vi "Initialize Stimulator_v0.vi"(4 "error in (no error)":errorcluster, 6 "Initialization Parameters":T6={"Stimulator Control"={"Name"="", "Mode"=enum."SIM", "Visa Timeout"=0}, "Initialization Parameters"={"Frequency"=0.0, "N Factor"=0, "D/T Int"=0.0, "Active Channels"=[TRUE, TRUE, TRUE, TRUE, TRUE], "LF Channels"=[FALSE, FALSE, FALSE, FALSE, FALSE]}}, 7 "Stimulator":T1={"Log File In"=refnum, "Stimulator In"="", "Stimulator Mode"="", "Log Data"=FALSE, "Doublet/Triplet  Interval"=0.0, "Stim Frequency"=0.0, "N-Factor"=0, "Active Channels"=[], "Low-Frequency Channels"=[], "Stimulator State"=enum."Closed", "Mode Array"=[], "Current Array"=[], "Pulse Duration Array"=[], "VISA Timeout"=50}) -> (0 "error out":errorcluster, 1 "Write to Log":string, 2 "Response":u8, 3 "Stimulator Out":T1={"Log File In"=refnum, "Stimulator In"="", "Stimulator Mode"="", "Log Data"=FALSE, "Doublet/Triplet  Interval"=0.0, "Stim Frequency"=40.0, "N-Factor"=0, "Active Channels"=[TRUE, TRUE, TRUE, TRUE, TRUE], "Low-Frequency Channels"=[FALSE, FALSE, FALSE, FALSE, FALSE], "Stimulator State"=enum."Closed", "Mode Array"=[], "Current Array"=[], "Pulse Duration Array"=[], "VISA Timeout"=50})   [LabVIEW 2019]
doc: "Use this template to build a VI to use as a subVI."
uses:
  Controls/Stimulator Cluster.ctl
  Controls/Stimulator Mode.ctl
  Version 2/Data Type Defs/Pulse Mode (array).ctl
  Controls/Stim Current Array.ctl
  Controls/Pulse Duration Array.ctl
  Version 2/Data Type Defs/Obsolete/Stimulator Init Control_obs.ctl
  Version 2/Data Type Defs/Stim Init Data.ctl
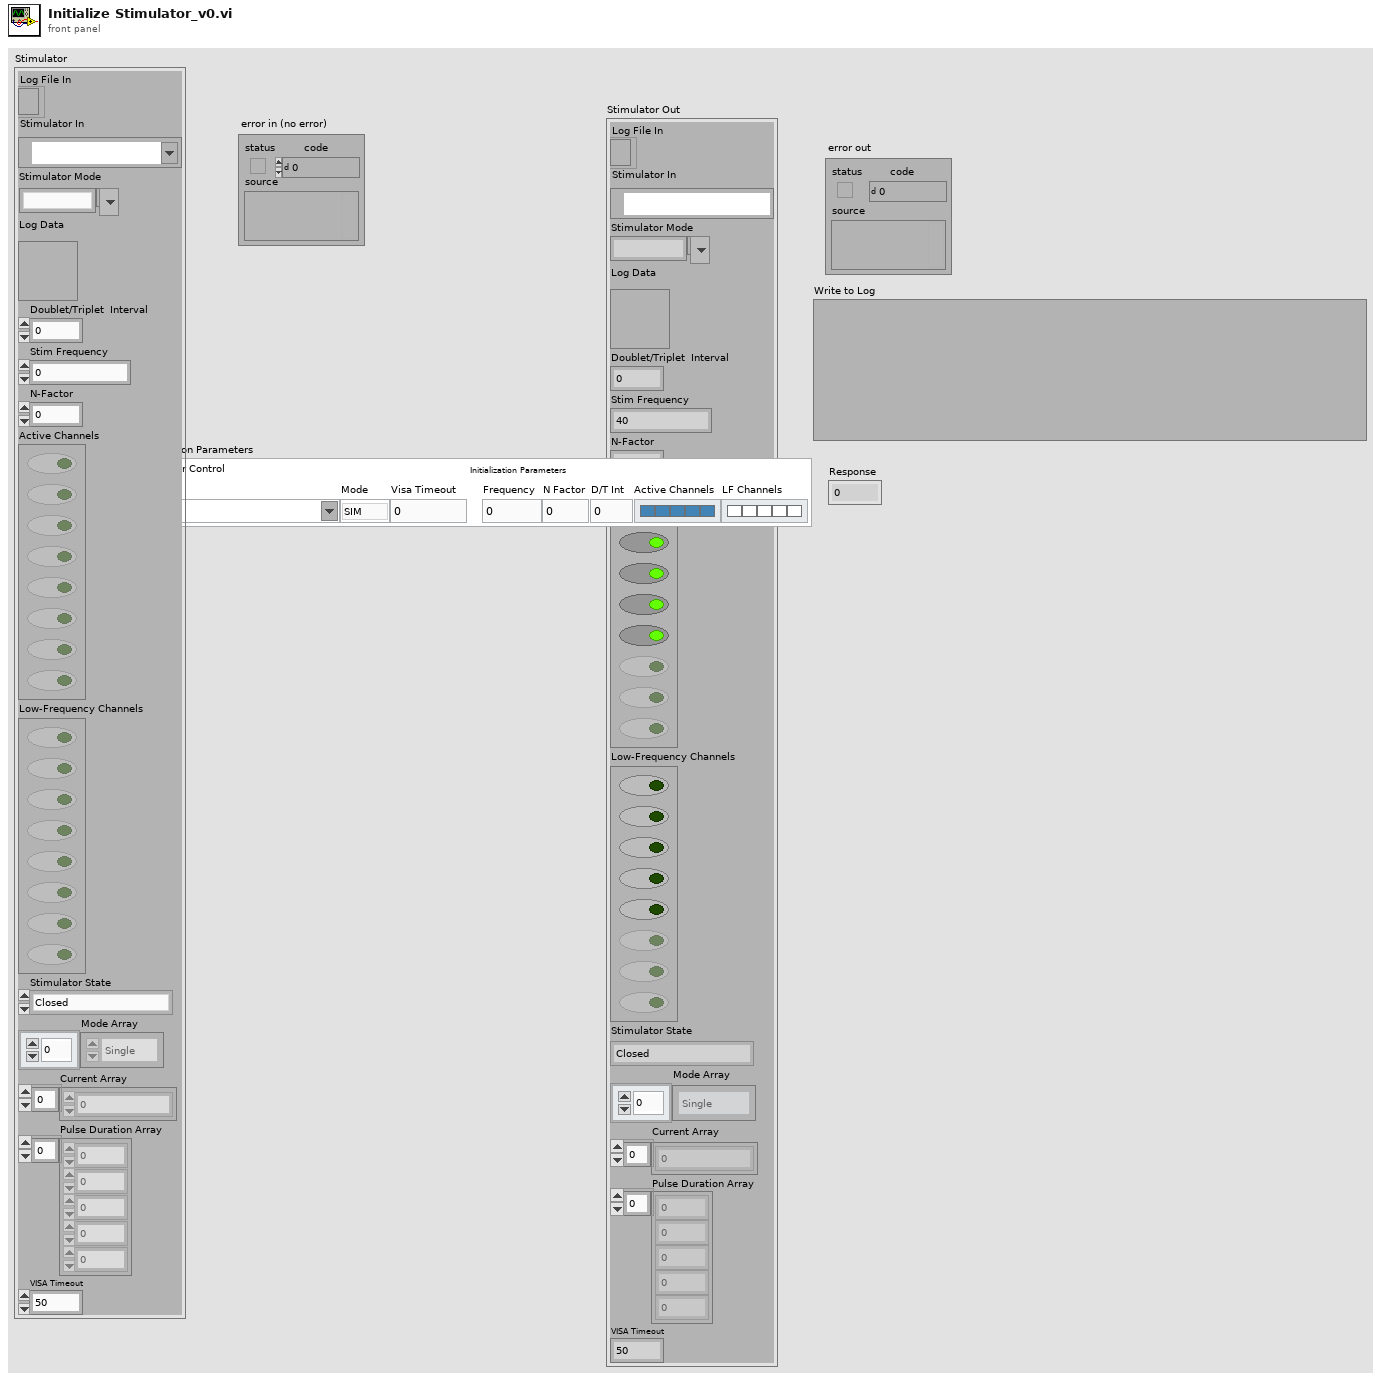
[diagram p1: front panel]
types:
  T1 = typedef "Stimulator Cluster.ctl" = cluster{"Log File In":refnum<file>, "Stimulator In":refnum<visa-resource-name>, "Stimulator Mode":T2, "Log Data":bool, "Doublet/Triplet  Interval":dbl, "Stim Frequency":dbl, "N-Factor":u8, "Active Channels":bool[], "Low-Frequency Channels":bool[], "Stimulator State":enum16{"Closed", "Open", "Initialized", "Stimulating"}, "Mode Array":T3, "Current Array":T4, "Pulse Duration Array":T5, "VISA Timeout":u32}
  T2 = typedef "Stimulator Mode.ctl" = string
  T3 = typedef "Pulse Mode (array).ctl" = enum16{"Single", "Doublet", "Triplet"}[]
  T4 = typedef "Stim Current Array.ctl" = u8[]
  T5 = typedef "Pulse Duration Array.ctl" = u32[]
  T6 = typedef "Stimulator Init Control_obs.ctl" = cluster{"Stimulator Control":cluster{"Name":refnum<visa-resource-name>, "Mode":enum16{"LIVE", "SIM"}, "Visa Timeout":u32}, "Initialization Parameters":T7}
  T7 = typedef "Stim Init Data.ctl" = cluster{"Frequency":dbl, "N Factor":u8, "D/T Int":dbl, "Active Channels":bool[], "LF Channels":bool[]}
  T8 = cluster{"Command Name":string, "Command String":string, "Log String":string}
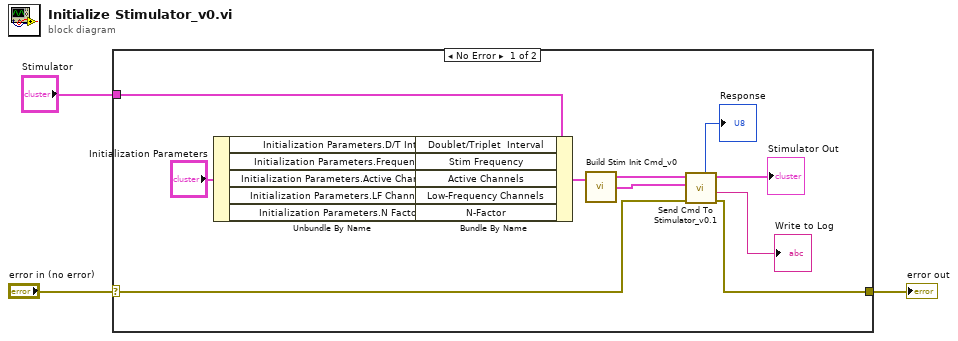
[diagram p0: block diagram]
diagram:
  n1 = case shown="No Error" "error in (no error)" {
    selector: "error in (no error)" -> [w5 w19]
    tunnel: [w4 w19] -> w2
    tunnel: "Stimulator" -> [w6 _]
    frame No Error {
      n2 = Unbundle By Name("Initialization Parameters") -> ("Initialization Parameters.D/T Int"=w13:dbl, "Initialization Parameters.Frequency"=w12:dbl, "Initialization Parameters.Active Channels"=w11:bool[], "Initialization Parameters.LF Channels"=w10:bool[], "Initialization Parameters.N Factor"=w9:u8)
      n3 = Bundle By Name(cluster=w6, "Doublet/Triplet  Interval"=w13, "Stim Frequency"=w12, "Active Channels"=w11, "Low-Frequency Channels"=w10, "N-Factor"=w9) -> (w18:T1)
      n4 = call "Build Stim Init Cmd_v0.vi"("Stimulator In"=w18) -> ("Stimulator Out"=w17:T1, "Command"=w15:T8)  [unwired: 2 in]
      n5 = call "Send Cmd To Stimulator_v0.1.vi"("Stimulator In"=w17, "Command"=w15, "error in (no error)"=w5) -> ("Numeric Response"=→"Response":u8, "Stimulator Out"=→"Stimulator Out":T1, "Log Entry"=→"Write to Log":string, "error out"=w4:errorcluster)  [unwired: 1 in, 1 out]
    }
    frame Error {
    }
  }
  "error out" <- w2
